vi "Display Image.vi"(0 "ImageHandler in":refnum<class "ImageHandler.lvclass">, 5 "Path":path, 7 "Image Indicator":refnum<vi>, 11 "error in (no error)":errorcluster) -> (4 "ImageHandler out":refnum<class "ImageHandler.lvclass">, 15 "error out":errorcluster)   [LabVIEW 2021, in "ImageHandler.lvlib" / "ImageHandler.lvclass"]
uses:
  ImageHandler.lvclass
  ImageHandler.lvclass/ImageHandler.ctl
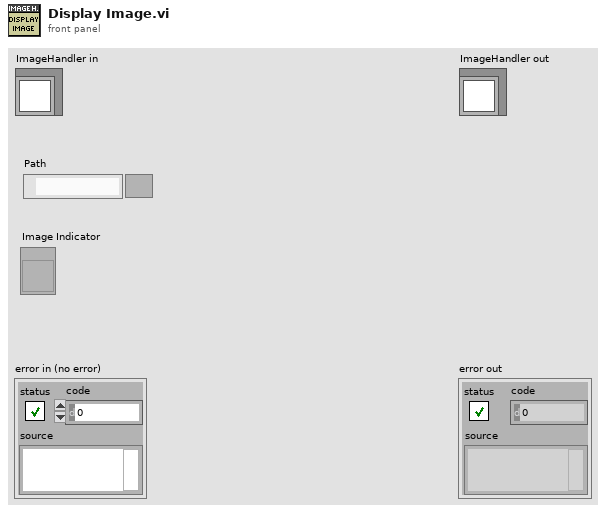
[diagram p1: front panel]
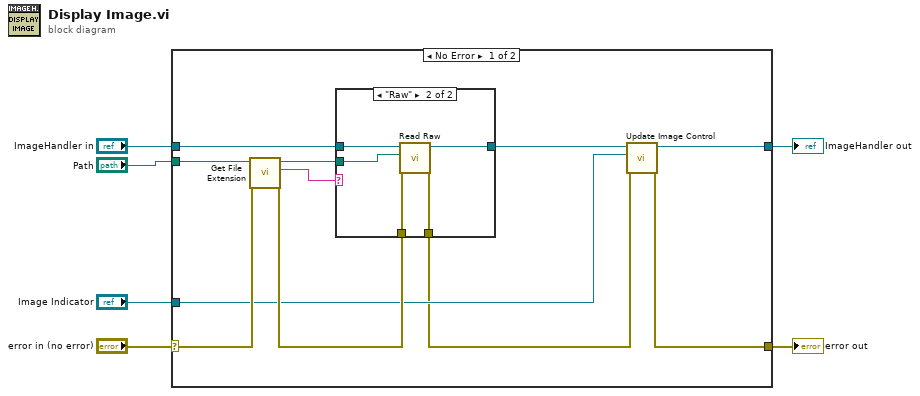
[diagram p0: block diagram]
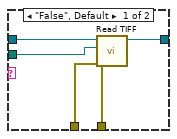
[diagram p2: hidden frame]
diagram:
  n1 = case shown="No Error" "error in (no error)" {
    selector: "error in (no error)" -> [w16 w29]
    tunnel: [w7 w29] -> w5
    tunnel: [w9 w28] -> w3
    tunnel: "ImageHandler in" -> [w12 w28]
    tunnel: "Path" -> [w17 _]
    tunnel: "Image Indicator" -> [w10 _]
    frame No Error {
      n2 = call <vilib>:"Get File Extension.vi"("error in (no error)"=w16, "file"=w17) -> ("error out"=w13:errorcluster, "lowercase file extension"=w15:string, "dup file"=w14:path)  [unwired: 5 in, 2 out]
      n3 = case shown="\"Raw\"" w15 {
        tunnel: w12 -> [w22 w27]
        tunnel: w14 -> [w18 w23]
        tunnel: [w21 w26] -> w11
        tunnel: w13 -> [w20 w25]
        tunnel: [w19 w24] -> w8
        frame "False", Default {
          n4 = call "Read TIFF.vi"("error in (no error)"=w20, "Path"=w18, "ImageHandler in"=w22) -> ("error out"=w19:errorcluster, "ImageHandler out"=w21:refnum<class "ImageHandler.lvclass">)  [unwired: 7 in]
        }
        frame "Raw" {
          n5 = call "Read Raw.vi"("error in (no error)"=w25, "Path"=w23, "ImageHandler in"=w27) -> ("error out"=w24:errorcluster, "ImageHandler out"=w26:refnum<class "ImageHandler.lvclass">)  [unwired: 7 in]
        }
      }
      n6 = call "Update Image Control.vi"("error in (no error)"=w8, "Image Indicator"=w10, "ImageHandler in"=w11) -> ("error out"=w7:errorcluster, "ImageHandler out"=w9:refnum<class "ImageHandler.lvclass">)  [unwired: 7 in]
    }
    frame Error {
    }
  }
  "error out" <- w5
  "ImageHandler out" <- w3
